vi "Split VIP File Name to Unique Name and Version.vi"(0 "VI Package File Name (with extension) in":path) -> (4 "Unique Name":string, 6 "Version":string)   [LabVIEW 2017, in "CL_G3_VIPMUtilities.lvlib"]
uses:
  CL_G3_VIPMUtilities.lvlib
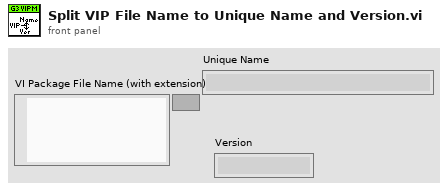
[diagram p1: front panel]
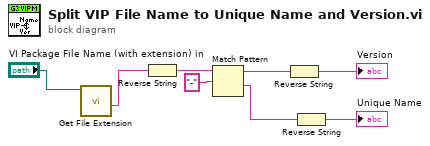
[diagram p0: block diagram]
diagram:
  n1 = call <vilib>:"Get File Extension.vi"("file"="VI Package File Name (with extension) in") -> ("filename without extension"=w1:string)  [unwired: 6 in, 4 out]
  n2 = Reverse String(1:w1) -> (0:w7:string)
  n3 = Match Pattern(string=w7, regular expression="-") -> (before substring=w6:string, after substring=w5:string)  [unwired: 1 in, 2 out]
  n4 = Reverse String(1:w6) -> (0:→"Version":string)
  n5 = Reverse String(1:w5) -> (0:→"Unique Name":string)
